vi "자판기 만들기 실습.vi"() -> ()   [LabVIEW 2020]
panel:
  in  "정지":bool
  in  "거스름돈 반환":bool
  out "배출 상품명":string
  out "현재잔액":dbl
  in  "1000원":bool
  in  "500원":bool
  in  "100원":bool
  in  "50원":bool
  in  "10원":bool
  out "웰치스 LED":bool
  out "콜라 LED":bool
  out "환타 LED":bool
  out "사이다 LED":bool
  in  "웰치스":bool
  in  "콜라":bool
  in  "환타":bool
  in  "사이다":bool
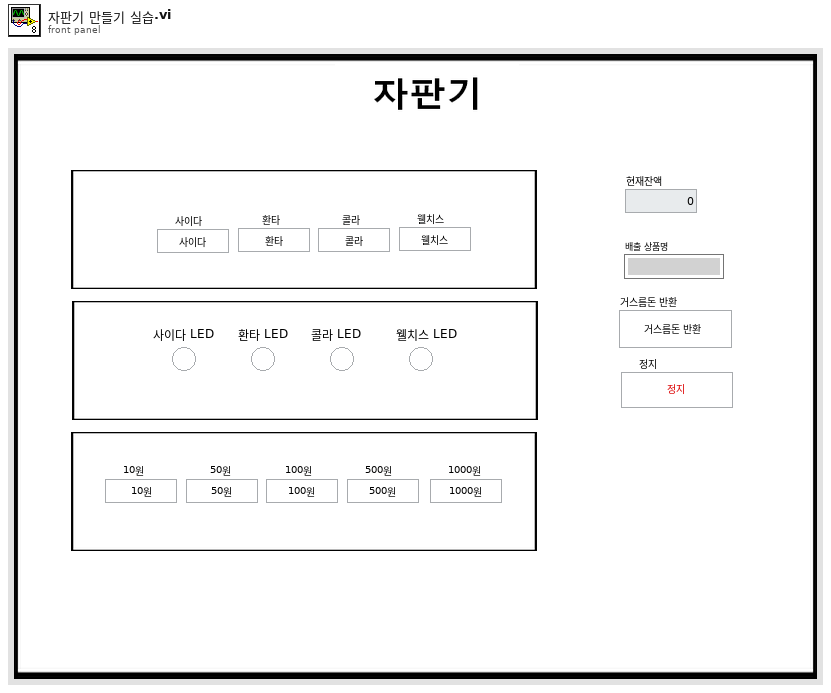
[diagram p1: front panel]
types:
  T1 = typedef "자판기 컨트롤.ctl" = enum16{"초기화", "10원", "50원", "100원", "500원", "1000원", "디스플레이 업데이트", "사이다", "콜라", "환타", "웰치스", "거스름돈 반환", "종료"}
  T2 = cluster{"사이다 LED":bool, "현재잔액":dbl, "웰치스 LED":bool, "환타 LED":bool, "콜라 LED":bool, "배출 상품명":string}
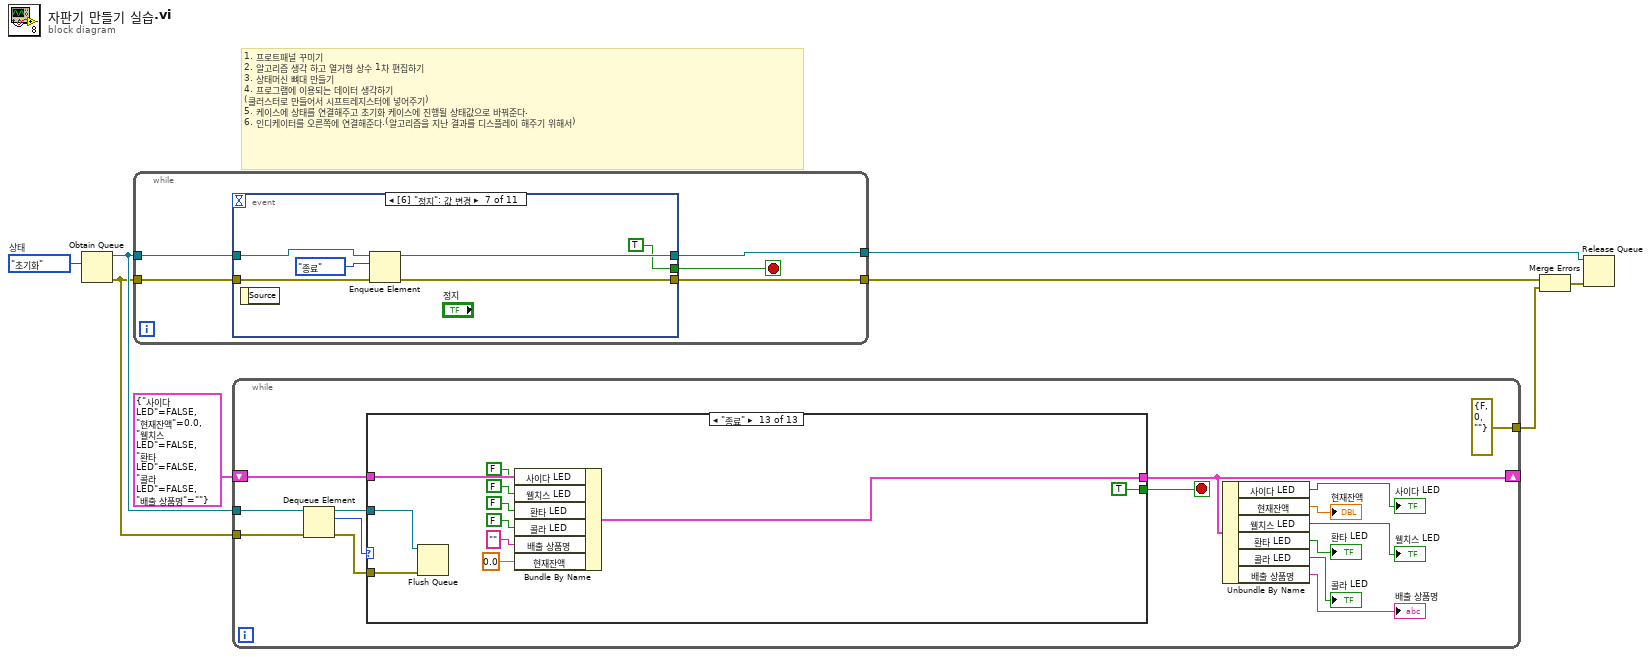
[diagram p0: block diagram]
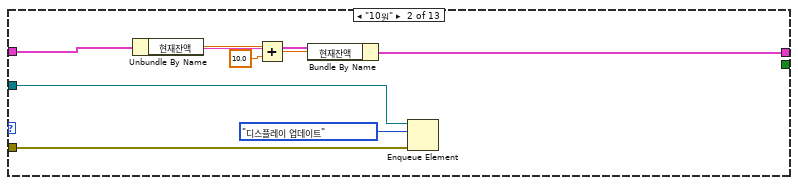
[diagram p3: hidden frame]
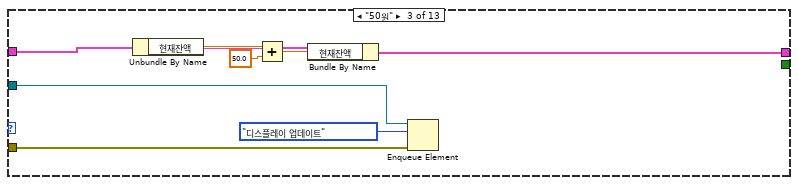
[diagram p4: hidden frame]
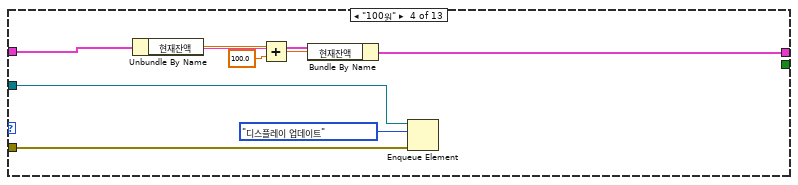
[diagram p5: hidden frame]
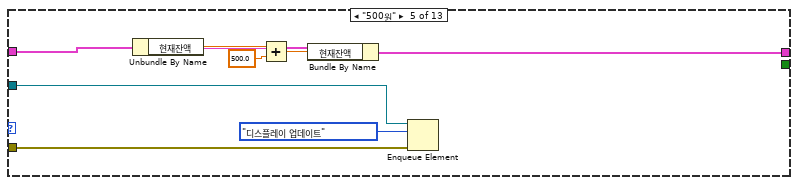
[diagram p6: hidden frame]
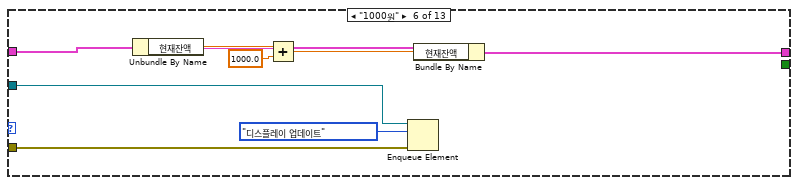
[diagram p7: hidden frame]
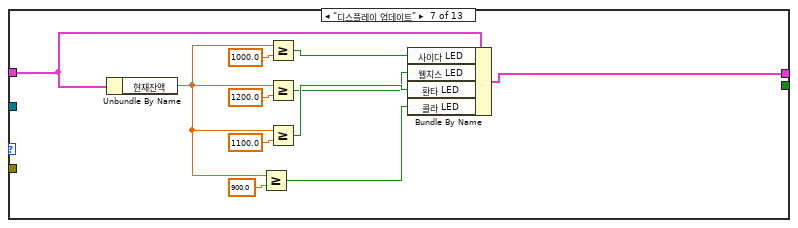
[diagram p8: hidden frame]
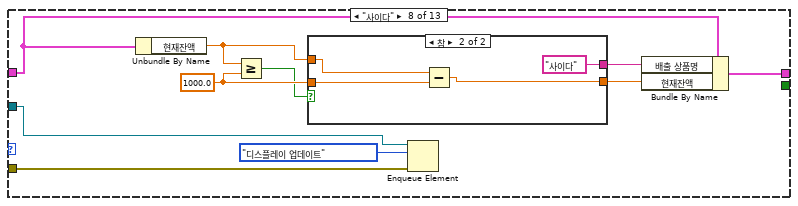
[diagram p9: hidden frame]
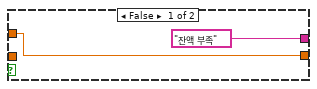
[diagram p10: hidden frame]
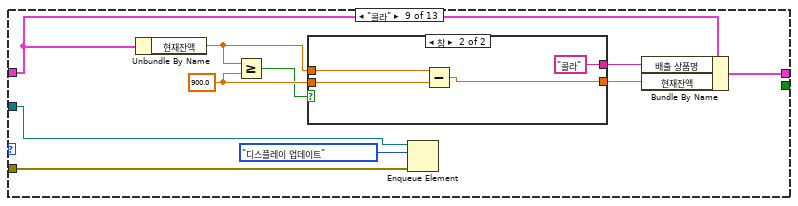
[diagram p11: hidden frame]
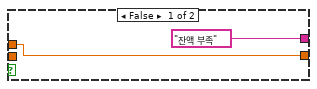
[diagram p12: hidden frame]
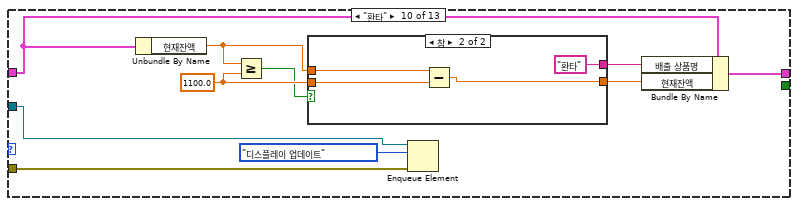
[diagram p13: hidden frame]
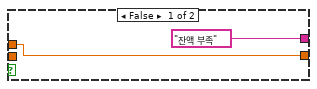
[diagram p14: hidden frame]
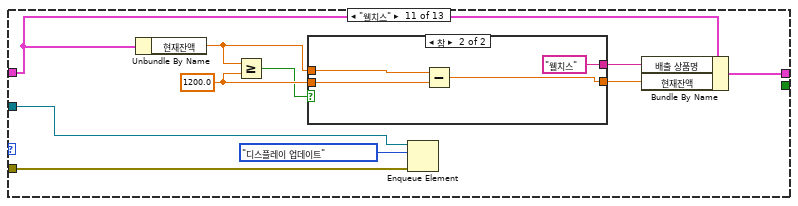
[diagram p15: hidden frame]
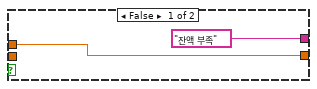
[diagram p16: hidden frame]
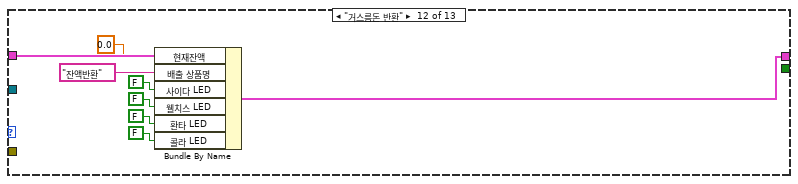
[diagram p17: hidden frame]
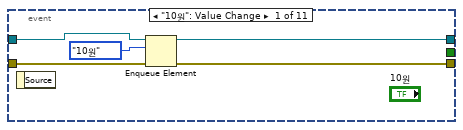
[diagram p18: hidden frame]
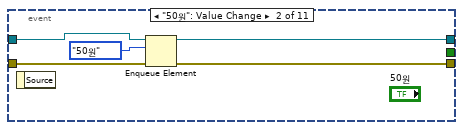
[diagram p19: hidden frame]
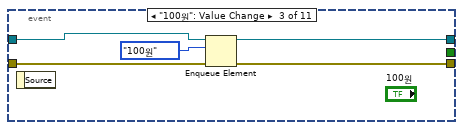
[diagram p20: hidden frame]
diagram:
  w8 = 자판기_컨트롤."초기화"  # 상태
  # "1. 프로트패널 꾸미기\n2. 알고리즘 생각 하고 열거형 상수 1차 편집하기\n3. 상태머신 뼈대 만들기\n4. 프로그램에 이용되는 데이터 생각하기\n(클러스터로 만들어서 시프트레지스터에 넣어주기)\n5. 케이스에 상태를 연결해주고 초기화 케이스에 진행될 상태값으로 바꿔준다.\n6. 인디케이터를 오른쪽에 연결해준다.(알고리즘을 지난 결과를 디스플레이 해주기 위해서)"
  n1 = Obtain Queue(element data type=w8) -> (queue out=w7:refnum<queue>, error out=w6:errorcluster)  [unwired: 4 in, 1 out]
  n2 = while {
    tunnel: w7 -> [w13]
    tunnel: w6 -> [w12]
    tunnel: [w11] -> w5
    tunnel: [w10] -> w2
    stop <- w9 stop-if-true
    n3 = event shown="[6] \"정지\": 값 변경" {
      selector: _ -> [_ _ _ _ _ _ _ _ _ _ _]
      dyn-events: _ -> [_ _ _ _ _ _ _ _ _ _ _]
      timeout: _ -> [_ _ _ _ _ _ _ _ _ _ _]
      tunnel: w13 -> [w18 w23 w28 w33 w38 w43 w49 w54 w59 w64 w69]
      tunnel: w12 -> [w17 w22 w27 w32 w37 w42 w48 w53 w58 w63 w68]
      tunnel: [w15 w20 w25 w30 w35 w40 w46 w51 w56 w61 w66] -> w11
      tunnel: [w14 w19 w24 w29 w34 w39 w45 w50 w55 w60 w65] -> w10
      tunnel: [_ _ _ _ _ _ TRUE _ _ _ _] -> w9
      event "10원": Value Change {
        n4 = event-data() -> ()  [unwired: 1 in, 1 out]
        n5 = Enqueue Element(queue=w18, element=자판기_컨트롤."10원" ("원소"), error in (no error)=w17) -> (queue out=w14:refnum<queue>, error out=w15:errorcluster)  [unwired: 1 in, 1 out]
      }
      event "50원": Value Change {
        n6 = event-data() -> ()  [unwired: 1 in, 1 out]
        n7 = Enqueue Element(queue=w23, element=자판기_컨트롤."50원" ("원소"), error in (no error)=w22) -> (queue out=w19:refnum<queue>, error out=w20:errorcluster)  [unwired: 1 in, 1 out]
      }
      event "100원": Value Change {
        n8 = event-data() -> ()  [unwired: 1 in, 1 out]
        n9 = Enqueue Element(queue=w28, element=자판기_컨트롤."100원" ("원소"), error in (no error)=w27) -> (queue out=w24:refnum<queue>, error out=w25:errorcluster)  [unwired: 1 in, 1 out]
      }
      event "500원": Value Change {
        n10 = event-data() -> ()  [unwired: 1 in, 1 out]
        n11 = Enqueue Element(queue=w33, element=자판기_컨트롤."500원" ("원소"), error in (no error)=w32) -> (queue out=w29:refnum<queue>, error out=w30:errorcluster)  [unwired: 1 in, 1 out]
      }
      event "1000원": Value Change {
        n12 = event-data() -> ()  [unwired: 1 in, 1 out]
        n13 = Enqueue Element(queue=w38, element=자판기_컨트롤."1000원" ("원소"), error in (no error)=w37) -> (queue out=w34:refnum<queue>, error out=w35:errorcluster)  [unwired: 1 in, 1 out]
      }
      event "거스름돈 반환": Value Change {
        n14 = event-data() -> ()  [unwired: 1 in, 1 out]
        n15 = Enqueue Element(queue=w43, element=자판기_컨트롤."거스름돈 반환" ("원소"), error in (no error)=w42) -> (queue out=w39:refnum<queue>, error out=w40:errorcluster)  [unwired: 1 in, 1 out]
      }
      event "정지": Value Change {
        n16 = event-data() -> ()  [unwired: 1 in, 1 out]
        n17 = Enqueue Element(queue=w49, element=자판기_컨트롤."종료" ("원소"), error in (no error)=w48) -> (queue out=w45:refnum<queue>, error out=w46:errorcluster)  [unwired: 1 in, 1 out]
      }
      event "사이다": Value Change {
        n18 = event-data() -> ()  [unwired: 1 in, 1 out]
        n19 = Enqueue Element(queue=w54, element=자판기_컨트롤."사이다" ("원소"), error in (no error)=w53) -> (queue out=w50:refnum<queue>, error out=w51:errorcluster)  [unwired: 1 in, 1 out]
      }
      event "환타": Value Change {
        n20 = event-data() -> ()  [unwired: 1 in, 1 out]
        n21 = Enqueue Element(queue=w59, element=자판기_컨트롤."환타" ("원소"), error in (no error)=w58) -> (queue out=w55:refnum<queue>, error out=w56:errorcluster)  [unwired: 1 in, 1 out]
      }
      event "콜라": Value Change {
        n22 = event-data() -> ()  [unwired: 1 in, 1 out]
        n23 = Enqueue Element(queue=w64, element=자판기_컨트롤."콜라" ("원소"), error in (no error)=w63) -> (queue out=w60:refnum<queue>, error out=w61:errorcluster)  [unwired: 1 in, 1 out]
      }
      event "웰치스": Value Change {
        n24 = event-data() -> ()  [unwired: 1 in, 1 out]
        n25 = Enqueue Element(queue=w69, element=자판기_컨트롤."웰치스" ("원소"), error in (no error)=w68) -> (queue out=w65:refnum<queue>, error out=w66:errorcluster)  [unwired: 1 in, 1 out]
      }
    }
  }
  n26 = while {
    tunnel: w7 -> [w84]
    tunnel: w6 -> [w83]
    tunnel: [errorcluster {"status"=FALSE, "code"=0, "source"=""} ("에러 상수")] -> w4
    shift-right: [w78] -> _
    shift-left: T2 {"사이다 LED"=FALSE, "현재잔액"=0.0, "웰치스 LED"=FALSE, "환타 LED"=FALSE, "콜라 LED"=FALSE, "배출 상품명"=""} -> [w80]
    stop <- w79 stop-if-true
    n27 = Dequeue Element(queue=w84, error in (no error)=w83) -> (queue out=w73:refnum<queue>, element=w82:T1, error out=w72:errorcluster)  [unwired: 1 in, 1 out]
    n28 = case shown="\"종료\"" w82 {
      tunnel: w80 -> [_ w90 w98 w106 w114 w122 w130 w140 w156 w172 w188 w207 w215]
      tunnel: [_ w88 w96 w104 w112 w120 w128 w139 w155 w171 w187 w204 w214] -> w78
      tunnel: [_ _ _ _ _ _ _ _ _ _ _ _ TRUE] -> w79
      tunnel: w73 -> [_ w86 w94 w102 w110 w119 _ w137 w153 w169 w185 _ w217]
      tunnel: w72 -> [_ w85 w93 w101 w109 w118 _ w136 w152 w168 w184 _ w216]
      frame "초기화", Default {
      }
      frame "10원" {
        n29 = Unbundle By Name(w90) -> ("현재잔액"=w91:dbl)
        n30 = Add(x=w91, y=10.0) -> (x+y=w89:dbl)
        n31 = Bundle By Name(cluster=w90, "현재잔액"=w89) -> (w88:T2)
        n32 = Enqueue Element(queue=w86, element=자판기_컨트롤."디스플레이 업데이트" ("원소"), error in (no error)=w85) -> ()  [unwired: 1 in, 3 out]
      }
      frame "50원" {
        n33 = Unbundle By Name(w98) -> ("현재잔액"=w99:dbl)
        n34 = Add(x=w99, y=50.0) -> (x+y=w97:dbl)
        n35 = Bundle By Name(cluster=w98, "현재잔액"=w97) -> (w96:T2)
        n36 = Enqueue Element(queue=w94, element=자판기_컨트롤."디스플레이 업데이트" ("원소"), error in (no error)=w93) -> ()  [unwired: 1 in, 3 out]
      }
      frame "100원" {
        n37 = Unbundle By Name(w106) -> ("현재잔액"=w107:dbl)
        n38 = Add(x=w107, y=100.0) -> (x+y=w105:dbl)
        n39 = Bundle By Name(cluster=w106, "현재잔액"=w105) -> (w104:T2)
        n40 = Enqueue Element(queue=w102, element=자판기_컨트롤."디스플레이 업데이트" ("원소"), error in (no error)=w101) -> ()  [unwired: 1 in, 3 out]
      }
      frame "500원" {
        n41 = Unbundle By Name(w114) -> ("현재잔액"=w115:dbl)
        n42 = Add(x=w115, y=500.0) -> (x+y=w113:dbl)
        n43 = Bundle By Name(cluster=w114, "현재잔액"=w113) -> (w112:T2)
        n44 = Enqueue Element(queue=w110, element=자판기_컨트롤."디스플레이 업데이트" ("원소"), error in (no error)=w109) -> ()  [unwired: 1 in, 3 out]
      }
      frame "1000원" {
        n45 = Unbundle By Name(w122) -> ("현재잔액"=w123:dbl)
        n46 = Add(x=w123, y=1000.0) -> (x+y=w121:dbl)
        n47 = Enqueue Element(queue=w119, element=자판기_컨트롤."디스플레이 업데이트" ("원소"), error in (no error)=w118) -> ()  [unwired: 1 in, 3 out]
        n48 = Bundle By Name(cluster=w122, "현재잔액"=w121) -> (w120:T2)
      }
      frame "디스플레이 업데이트" {
        n49 = Unbundle By Name(w130) -> ("현재잔액"=w131:dbl)
        n50 = Greater Or Equal?(x=w131, y=900.0) -> (x >= y?=w127:bool)
        n51 = Greater Or Equal?(x=w131, y=1000.0) -> (x >= y?=w129:bool)
        n52 = Greater Or Equal?(x=w131, y=1200.0) -> (x >= y?=w125:bool)
        n53 = Greater Or Equal?(x=w131, y=1100.0) -> (x >= y?=w126:bool)
        n54 = Bundle By Name(cluster=w130, "사이다 LED"=w129, "웰치스 LED"=w125, "환타 LED"=w126, "콜라 LED"=w127) -> (w128:T2)
      }
      frame "사이다" {
        w144 = 1000.0 ("y")
        n55 = Unbundle By Name(w140) -> ("현재잔액"=w143:dbl)
        n56 = Greater Or Equal?(x=w143, y=w144) -> (x >= y?=w141:bool)
        n57 = case shown="참" w141 {
          tunnel: ["잔액 부족" "사이다"] -> w142
          tunnel: w143 -> [w146 w150]
          tunnel: w144 -> [_ w149]
          tunnel: [w146 w148] -> w145
          frame False {
          }
          frame True {
            n58 = Subtract(x=w150, y=w149) -> (x-y=w148:dbl)
          }
        }
        n59 = Enqueue Element(queue=w137, element=자판기_컨트롤."디스플레이 업데이트" ("원소"), error in (no error)=w136) -> ()  [unwired: 1 in, 3 out]
        n60 = Bundle By Name(cluster=w140, "배출 상품명"=w142, "현재잔액"=w145) -> (w139:T2)
      }
      frame "콜라" {
        w160 = 900.0 ("y")
        n61 = Unbundle By Name(w156) -> ("현재잔액"=w159:dbl)
        n62 = Greater Or Equal?(x=w159, y=w160) -> (x >= y?=w157:bool)
        n63 = case shown="참" w157 {
          tunnel: ["잔액 부족" "콜라"] -> w158
          tunnel: w159 -> [w162 w166]
          tunnel: w160 -> [_ w165]
          tunnel: [w162 w164] -> w161
          frame False {
          }
          frame True {
            n64 = Subtract(x=w166, y=w165) -> (x-y=w164:dbl)
          }
        }
        n65 = Enqueue Element(queue=w153, element=자판기_컨트롤."디스플레이 업데이트" ("원소"), error in (no error)=w152) -> ()  [unwired: 1 in, 3 out]
        n66 = Bundle By Name(cluster=w156, "배출 상품명"=w158, "현재잔액"=w161) -> (w155:T2)
      }
      frame "환타" {
        w176 = 1100.0 ("y")
        n67 = Unbundle By Name(w172) -> ("현재잔액"=w175:dbl)
        n68 = Greater Or Equal?(x=w175, y=w176) -> (x >= y?=w173:bool)
        n69 = case shown="참" w173 {
          tunnel: ["잔액 부족" "환타"] -> w174
          tunnel: w175 -> [w178 w182]
          tunnel: w176 -> [_ w181]
          tunnel: [w178 w180] -> w177
          frame False {
          }
          frame True {
            n70 = Subtract(x=w182, y=w181) -> (x-y=w180:dbl)
          }
        }
        n71 = Enqueue Element(queue=w169, element=자판기_컨트롤."디스플레이 업데이트" ("원소"), error in (no error)=w168) -> ()  [unwired: 1 in, 3 out]
        n72 = Bundle By Name(cluster=w172, "배출 상품명"=w174, "현재잔액"=w177) -> (w171:T2)
      }
      frame "웰치스" {
        w192 = 1200.0 ("y")
        n73 = Unbundle By Name(w188) -> ("현재잔액"=w191:dbl)
        n74 = Greater Or Equal?(x=w191, y=w192) -> (x >= y?=w189:bool)
        n75 = case shown="참" w189 {
          tunnel: ["잔액 부족" "웰치스"] -> w190
          tunnel: w191 -> [w194 w198]
          tunnel: w192 -> [_ w197]
          tunnel: [w194 w196] -> w193
          frame False {
          }
          frame True {
            n76 = Subtract(x=w198, y=w197) -> (x-y=w196:dbl)
          }
        }
        n77 = Enqueue Element(queue=w185, element=자판기_컨트롤."디스플레이 업데이트" ("원소"), error in (no error)=w184) -> ()  [unwired: 1 in, 3 out]
        n78 = Bundle By Name(cluster=w188, "배출 상품명"=w190, "현재잔액"=w193) -> (w187:T2)
      }
      frame "거스름돈 반환" {
        n79 = Bundle By Name(cluster=w207, "현재잔액"=0.0, "배출 상품명"="잔액반환", "사이다 LED"=FALSE, "웰치스 LED"=FALSE, "환타 LED"=FALSE, "콜라 LED"=FALSE) -> (w204:T2)
      }
      frame "종료" {
        n80 = Flush Queue(queue=w217, error in (no error)=w216) -> ()  [unwired: 3 out]
        n81 = Bundle By Name(cluster=w215, "사이다 LED"=FALSE, "웰치스 LED"=FALSE, "환타 LED"=FALSE, "콜라 LED"=FALSE, "배출 상품명"="", "현재잔액"=0.0) -> (w214:T2)
      }
    }
    n82 = Unbundle By Name(w78) -> ("사이다 LED"=→"사이다 LED":bool, "현재잔액"=→"현재잔액":dbl, "웰치스 LED"=→"웰치스 LED":bool, "환타 LED"=→"환타 LED":bool, "콜라 LED"=→"콜라 LED":bool, "배출 상품명"=→"배출 상품명":string)
  }
  n83 = Merge Errors(w5, w4) -> (w3:errorcluster)
  n84 = Release Queue(queue=w2, error in (no error)=w3) -> ()  [unwired: 1 in, 3 out]
